vi "VIR.vi"(8 "Stopp":bool, 10 "SLOT":i32=100 min=0 max=999 step=100, 11 "USB":i32) -> ()   [LabVIEW 2020]
doc: "This VI provides a GUI for SLM modules. It implements an abstract module interface, where callers provide the only necessary and sufficient information for callee modules via the datafields USB, SLOT and Stopp. All module intern information are handled hidden by the module. Thereby, a caller must not \"know\" about such internals."
panel:
  in  "Trigger Level":dbl caption="Trigger Level [V]"
  in  "Trigger Source":u16(ring) items=["80 MHz (int.)", "40 MHz (int.)", "20 MHz (int.)", "10 MHz (int.)", " 5 MHz (int.)", " 2.5 MHz (int.)", "rising  edge (ext.)", "falling edge (ext.)"]
  in  "Fan Running":bool
  in  "ZeroBtn":bool caption="Boolean"
  in  "Pulsed Mode":bool
  in  "Intensity":sgl min=0 max=100 step=1 format="%.1f"
  out "Device Type":string
  in  "Frequency":u16(ring) items=["80 MHz (int.)", "40 MHz (int.)", "20 MHz (int.)", "10 MHz (int.)", " 5 MHz (int.)", " 2.5 MHz (int.)", "rising  edge (ext.)", "falling edge (ext.)"]
  # "%"
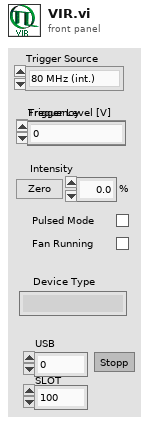
[diagram p1: front panel]
types:
  T1 = enum8{"Enabled", "Disabled", "Disabled and Grayed Out"}
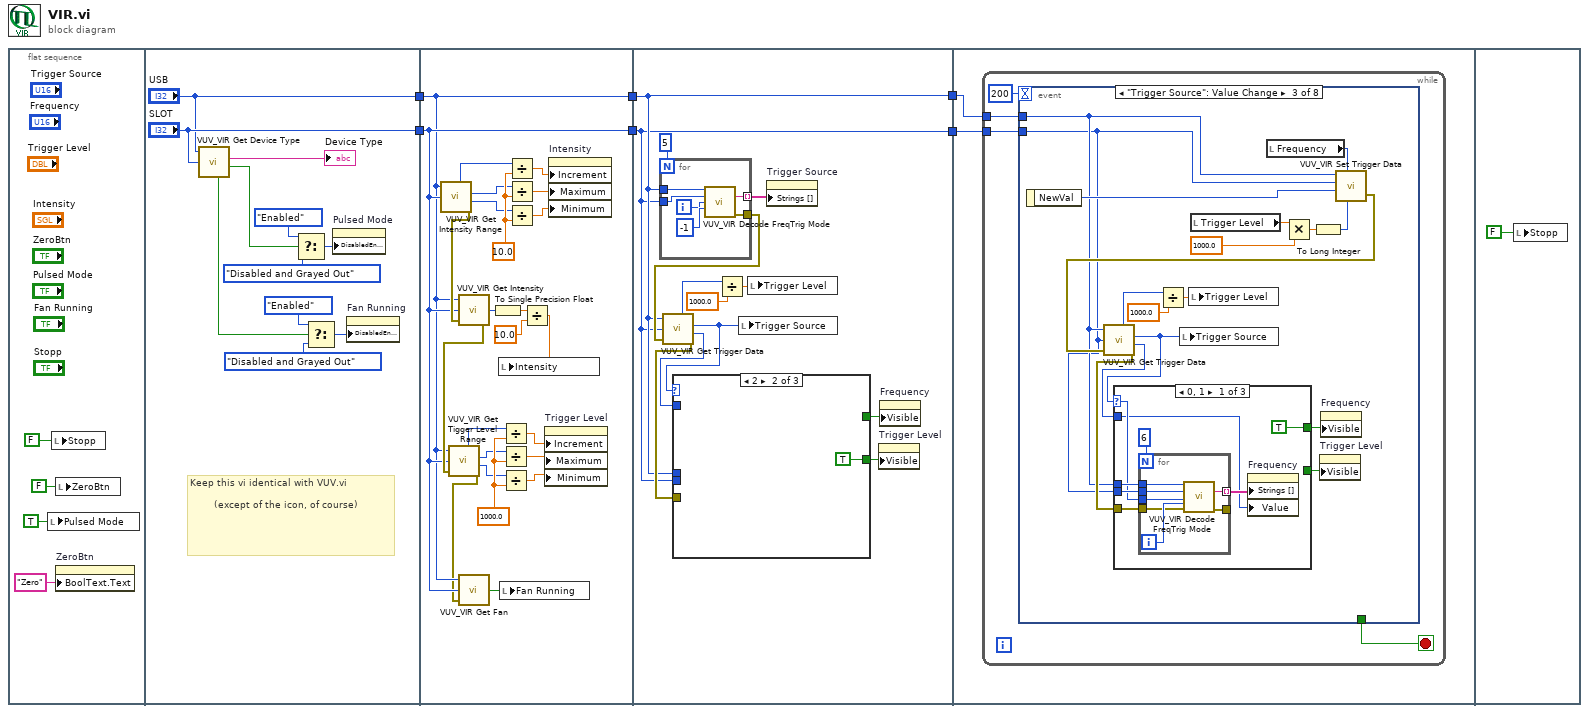
[diagram p0: block diagram]
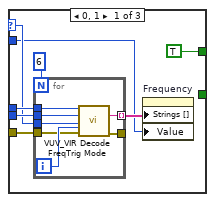
[diagram p2: hidden frame]
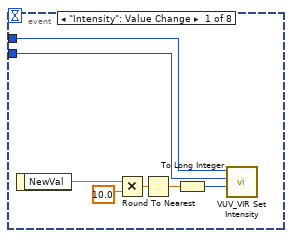
[diagram p4: hidden frame]
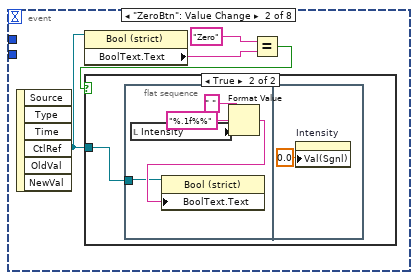
[diagram p5: hidden frame]
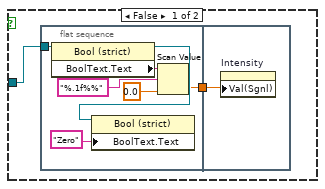
[diagram p6: hidden frame]
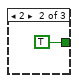
[diagram p7: hidden frame]
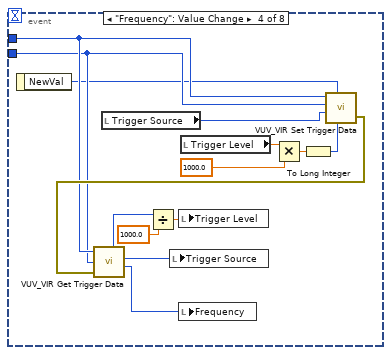
[diagram p9: hidden frame]
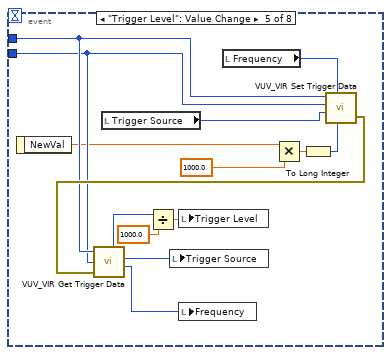
[diagram p10: hidden frame]
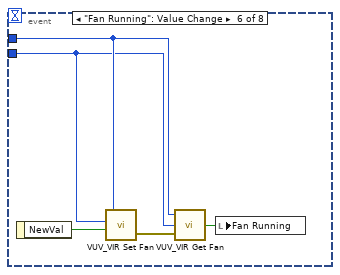
[diagram p11: hidden frame]
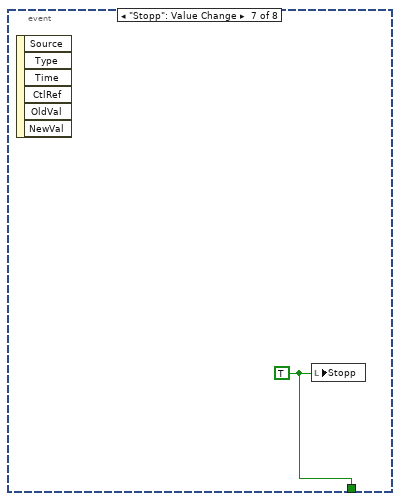
[diagram p12: hidden frame]
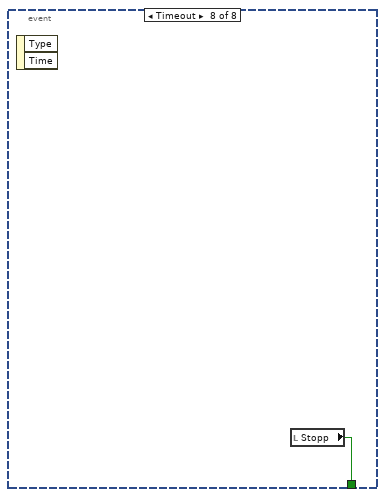
[diagram p13: hidden frame]
diagram:
  n1 = flat-sequence {
    tunnel: ["USB"] -> w6
    tunnel: ["SLOT"] -> w5
    tunnel: w6 -> [w24]
    tunnel: [w24] -> w4
    tunnel: w5 -> [w25]
    tunnel: [w25] -> w3
    tunnel: w4 -> [w47]
    tunnel: w3 -> [w46]
    tunnel: [w47] -> w2
    tunnel: [w46] -> w1
    tunnel: w2 -> [w81]
    tunnel: w1 -> [w82]
    frame #0 {
      n2 = local write "Pulsed Mode"(TRUE ("Pulsed Mode")) -> ()
      n3 = local write "Stopp"(FALSE ("Stopp")) -> ()
      n4 = local write "ZeroBtn"(FALSE ("ZeroBtn")) -> ()
      n5 = property on="ZeroBtn" class="Bool (strict)"("BoolText.Text"="Zero" ("Boolean Text.Text")) -> ()  [unwired: 2 in, 2 out]
    }
    frame #1 {
      # "Keep this vi identical with VUV.vi\n\n        (except of the icon, of course)"
      n6 = call "VUV_VIR Get Device Type.vi"("DevIdx"="USB", "SlotId"="SLOT") -> ("DeviceType"=→"Device Type":string, "OptCW"=w21:bool, "OptFanSwitch"=w14:bool)  [unwired: 1 in, 2 out]
      n7 = Select(t=T1."Enabled" ("Disabled"), s=w21, f=T1."Disabled and Grayed Out" ("Disabled")) -> (s? t:f=w18:T1)
      n8 = Select(t=T1."Enabled" ("Disabled"), s=w14, f=T1."Disabled and Grayed Out" ("Disabled")) -> (s? t:f=w15:T1)
      n9 = property on="Pulsed Mode" class="Bool (strict)"("DisabledEnum"=w18) -> ()  [unwired: 2 in, 2 out]
      n10 = property on="Fan Running" class="Bool (strict)"("DisabledEnum"=w15) -> ()  [unwired: 2 in, 2 out]
    }
    frame #2 {
      w30 = 1000.0
      w45 = 10.0
      n11 = call "VUV_VIR Get Intensity Range.vi"("DevIdx"=w24, "SlotId"=w25) -> ("UpperIntens"=w44:i32, "LowerIntens"=w42:i32, "error out"=w34:errorcluster, "ResolIntens"=w40:i32)  [unwired: 1 in, 1 out]
      n12 = call "VUV_VIR Get Intensity.vi"("error in (no error)"=w34, "SlotId"=w25, "DevIdx"=w24) -> ("error out"=w33:errorcluster, "Intensity"=w38:i32)  [unwired: 1 out]
      n13 = call "VUV_VIR Get Tigger Level Range.vi"("DevIdx"=w24, "SlotId"=w25, "error in (no error)"=w33) -> ("UpperTL"=w28:i32, "LowerTL"=w27:i32, "error out"=w23:errorcluster, "ResolTL"=w29:i32)  [unwired: 1 out]
      n14 = call "VUV_VIR Get Fan.vi"("error in (no error)"=w23, "SlotId"=w25, "DevIdx"=w24) -> ("FanRunning"=w26:bool)  [unwired: 2 out]
      n15 = To Single Precision Float(number=w38) -> (single precision float=w36:sgl)
      n16 = local write "Fan Running"(w26) -> ()
      n17 = Divide(x=w29, y=w30) -> (x/y=w32:dbl)
      n18 = Divide(x=w28, y=w30) -> (x/y=w31:dbl)
      n19 = Divide(x=w27, y=w30) -> (x/y=w22:dbl)
      n20 = Divide(x=w40, y=w45) -> (x/y=w39:dbl)
      n21 = Divide(x=w44, y=w45) -> (x/y=w43:dbl)
      n22 = Divide(x=w42, y=w45) -> (x/y=w41:dbl)
      n23 = Divide(x=w36, y=sgl 10.0) -> (x/y=w37:sgl)
      n24 = local write "Intensity"(w37) -> ()
      n25 = property on="Trigger Level" class="DigNum (strict)"("Increment"=w32, "Maximum"=w31, "Minimum"=w22) -> ()  [unwired: 2 in, 2 out]
      n26 = property on="Intensity" class="DigNum (strict)"("Increment"=w39, "Maximum"=w43, "Minimum"=w41) -> ()  [unwired: 2 in, 2 out]
    }
    frame #3 {
      n27 = for {
        N: 5 ("Numeric") -> [_]
        tunnel: w47 -> [w80]
        tunnel: w46 -> [w79]
        tunnel: [w76] -> w57 mode=indexing
        tunnel: [w75] -> w56
        i -> [w77]
        n28 = call "VUV_VIR Decode FreqTrig Mode.vi"("DevIdx"=w80, "SlotId"=w79, "MainTrigSrcIdx"=w77, "MainFreqDivIdx"=-1) -> ("MainFreqTrig"=w76:string, "error out"=w75:errorcluster)  [unwired: 6 in, 4 out]
      }
      n29 = call "VUV_VIR Get Trigger Data.vi"("DevIdx"=w47, "SlotId"=w46, "error in (no error)"=w56) -> ("MainTrigSrcIdx"=w54:i32, "MainFreqDivIdx"=w52:i32, "error out"=w55:errorcluster, "TrigLevel"=w51:i32)  [unwired: 1 out]
      n30 = case shown="2" w54 {
        selector: w54 -> [w62 _ _]
        tunnel: w47 -> [w65 _ _]
        tunnel: w46 -> [w64 _ _]
        tunnel: w55 -> [w63 _ _]
        tunnel: [TRUE _ _] -> w53
        tunnel: w52 -> [w59 _ _]
        tunnel: [_ TRUE _] -> w48
        frame 0, 1 {
          n31 = for {
            N: 6 ("Numeric") -> [_]
            tunnel: w65 -> [w73]
            tunnel: w64 -> [w72]
            tunnel: [w71] -> w61 mode=indexing
            tunnel: [w70] -> _
            tunnel: w63 -> [w68]
            tunnel: w62 -> [w67]
            i -> [w69]
            n32 = call "VUV_VIR Decode FreqTrig Mode.vi"("DevIdx"=w73, "SlotId"=w72, "MainTrigSrcIdx"=w67, "MainFreqDivIdx"=w69, "error in (no error)"=w68) -> ("MainFreqTrig"=w71:string, "error out"=w70:errorcluster)  [unwired: 5 in, 4 out]
          }
          n33 = property on="Frequency" class="Ring (strict)"("Strings []"=w61, "Value"=w59) -> ()  [unwired: 2 in, 2 out]
        }
        frame 2 {
        }
        frame Default {
        }
      }
      n34 = Divide(x=w51, y=1000.0) -> (x/y=w50:dbl)
      n35 = local write "Trigger Source"(w54) -> ()
      n36 = local write "Trigger Level"(w50) -> ()
      n37 = property on="Trigger Source" class="Ring (strict)"("Strings []"=w57) -> ()  [unwired: 2 in, 2 out]
      n38 = property on="Trigger Level" class="DigNum (strict)"("Visible"=w48) -> ()  [unwired: 2 in, 2 out]
      n39 = property on="Frequency" class="Ring (strict)"("Visible"=w53) -> ()  [unwired: 2 in, 2 out]
    }
    frame #4 {
      n40 = while {
        tunnel: w82 -> [w86]
        tunnel: w81 -> [w85]
        stop <- w83 stop-if-true
        n41 = event shown="[2] \"Trigger Source\": Value Change" {
          selector: _ -> [_ _ _ _ _ _ _ _]
          dyn-events: _ -> [_ _ _ _ _ _ _ _]
          timeout: 200 -> [_ _ _ _ _ _ _ _]
          tunnel: w86 -> [w88 _ w115 w151 w166 w176 _ _]
          tunnel: w85 -> [w87 _ w116 w152 w167 w177 _ _]
          tunnel: [_ _ _ _ _ _ w181 w182] -> w83
          event "Intensity": Value Change {
            n42 = event-data() -> ("NewVal"=w89:sgl)  [unwired: 1 in]
            n43 = Multiply(x=w89, y=sgl 10.0) -> (x*y=w93:sgl)
            n44 = Round To Nearest(number=w93) -> (nearest integer value=w91:sgl)
            n45 = To Long Integer(number=w91) -> (32bit integer=w92:i32)
            n46 = call "VUV_VIR Set Intensity.vi"("Intensity"=w92, "SlotId"=w88, "DevIdx"=w87) -> ()  [unwired: 1 in, 2 out]
          }
          event "ZeroBtn": Value Change {
            n47 = event-data() -> ("CtlRef"=w94:refnum<vi>)  [unwired: 1 in, 5 out]
            n48 = property class="Bool (strict)"(reference=w94) -> ("BoolText.Text"=w96:string)  [unwired: 1 in, 2 out]
            n49 = Equal?(x="Zero" ("Boolean Text.Text"), y=w96) -> (x = y?=w95:bool)
            n50 = case shown="True" w95 {
              tunnel: w94 -> [w99 w108]
              frame False {
                n51 = flat-sequence {
                  tunnel: w99 -> [w106]
                  tunnel: [w101] -> w98
                  tunnel: w98 -> [w107]
                  frame #0 {
                    n52 = property class="Bool (strict)"(reference=w106) -> (reference out=w103:refnum<vi>, "BoolText.Text"=w105:string)  [unwired: 1 in, 1 out]
                    n53 = property class="Bool (strict)"(reference=w103, "BoolText.Text"="Zero" ("Boolean Text.Text")) -> ()  [unwired: 1 in, 2 out]
                    n54 = Scan Value(string=w105, format string="%.1f%%", default (0 dbl)=0.0) -> (value=w101:dbl)  [unwired: 1 out]
                  }
                  frame #1 {
                    n55 = property on="Intensity" class="DigNum (strict)"("Val(Sgnl)"=w107) -> ()  [unwired: 2 in, 2 out]
                  }
                }
              }
              frame True {
                n56 = flat-sequence {
                  tunnel: w108 -> [w109]
                  frame #0 {
                    n57 = local read "Intensity"() -> (w111:sgl)
                    n58 = Format Value(string ("")=" ", format string="%.1f%%", value (0)=w111) -> (output string=w110:string)
                    n59 = property class="Bool (strict)"(reference=w109, "BoolText.Text"=w110) -> ()  [unwired: 1 in, 2 out]
                  }
                  frame #1 {
                    n60 = property on="Intensity" class="DigNum (strict)"("Val(Sgnl)"=sgl 0.0 ("Intensity")) -> ()  [unwired: 2 in, 2 out]
                  }
                }
              }
            }
          }
          event "Trigger Source": Value Change {
            n61 = event-data() -> ("NewVal"=w131:u16)  [unwired: 1 in]
            n62 = local read "Trigger Level"() -> (w129:dbl)
            n63 = local read "Frequency"() -> (w130:u16)
            n64 = Multiply(x=w129, y=1000.0) -> (x*y=w127:dbl)
            n65 = To Long Integer(number=w127) -> (32bit integer=w126:i32)
            n66 = call "VUV_VIR Set Trigger Data.vi"("TrigLevel"=w126, "MainFreqDivIdx"=w130, "MainTrigSrcIdx"=w131, "SlotId"=w115, "DevIdx"=w116) -> ("error out"=w119:errorcluster)  [unwired: 1 in, 1 out]
            n67 = call "VUV_VIR Get Trigger Data.vi"("DevIdx"=w116, "SlotId"=w115, "error in (no error)"=w119) -> ("MainTrigSrcIdx"=w120:i32, "MainFreqDivIdx"=w117:i32, "error out"=w118:errorcluster, "TrigLevel"=w122:i32)  [unwired: 1 out]
            n68 = case shown="0, 1" w120 {
              selector: w120 -> [w135 _ _]
              tunnel: w116 -> [w138 _ _]
              tunnel: w115 -> [w137 _ _]
              tunnel: w118 -> [w136 _ _]
              tunnel: [TRUE _ _] -> w121
              tunnel: w117 -> [w132 _ _]
              tunnel: [_ TRUE _] -> w125
              frame 0, 1 {
                n69 = for {
                  N: 6 ("Numeric") -> [_]
                  tunnel: w138 -> [w146]
                  tunnel: w137 -> [w145]
                  tunnel: [w144] -> w134 mode=indexing
                  tunnel: [w143] -> _
                  tunnel: w136 -> [w141]
                  tunnel: w135 -> [w140]
                  i -> [w142]
                  n70 = call "VUV_VIR Decode FreqTrig Mode.vi"("DevIdx"=w146, "SlotId"=w145, "MainTrigSrcIdx"=w140, "MainFreqDivIdx"=w142, "error in (no error)"=w141) -> ("MainFreqTrig"=w144:string, "error out"=w143:errorcluster)  [unwired: 5 in, 4 out]
                }
                n71 = property on="Frequency" class="Ring (strict)"("Strings []"=w134, "Value"=w132) -> ()  [unwired: 2 in, 2 out]
              }
              frame 2 {
              }
              frame Default {
              }
            }
            n72 = Divide(x=w122, y=1000.0) -> (x/y=w123:dbl)
            n73 = local write "Trigger Source"(w120) -> ()
            n74 = local write "Trigger Level"(w123) -> ()
            n75 = property on="Trigger Level" class="DigNum (strict)"("Visible"=w125) -> ()  [unwired: 2 in, 2 out]
            n76 = property on="Frequency" class="Ring (strict)"("Visible"=w121) -> ()  [unwired: 2 in, 2 out]
          }
          event "Frequency": Value Change {
            n77 = event-data() -> ("NewVal"=w150:u16)  [unwired: 1 in]
            n78 = local read "Trigger Source"() -> (w149:u16)
            n79 = local read "Trigger Level"() -> (w161:dbl)
            n80 = Multiply(x=w161, y=1000.0) -> (x*y=w159:dbl)
            n81 = To Long Integer(number=w159) -> (32bit integer=w158:i32)
            n82 = call "VUV_VIR Set Trigger Data.vi"("TrigLevel"=w158, "MainFreqDivIdx"=w150, "MainTrigSrcIdx"=w149, "SlotId"=w151, "DevIdx"=w152) -> ("error out"=w153:errorcluster)  [unwired: 1 in, 1 out]
            n83 = call "VUV_VIR Get Trigger Data.vi"("DevIdx"=w152, "SlotId"=w151, "error in (no error)"=w153) -> ("MainTrigSrcIdx"=w154:i32, "MainFreqDivIdx"=w148:i32, "TrigLevel"=w155:i32)  [unwired: 2 out]
            n84 = Divide(x=w155, y=1000.0) -> (x/y=w156:dbl)
            n85 = local write "Trigger Source"(w154) -> ()
            n86 = local write "Trigger Level"(w156) -> ()
            n87 = local write "Frequency"(w148) -> ()
          }
          event "Trigger Level": Value Change {
            n88 = event-data() -> ("NewVal"=w163:dbl)  [unwired: 1 in]
            n89 = local read "Trigger Source"() -> (w165:u16)
            n90 = local read "Frequency"() -> (w162:u16)
            n91 = Multiply(x=w163, y=1000.0) -> (x*y=w174:dbl)
            n92 = To Long Integer(number=w174) -> (32bit integer=w173:i32)
            n93 = call "VUV_VIR Set Trigger Data.vi"("TrigLevel"=w173, "MainFreqDivIdx"=w162, "MainTrigSrcIdx"=w165, "SlotId"=w166, "DevIdx"=w167) -> ("error out"=w168:errorcluster)  [unwired: 1 in, 1 out]
            n94 = call "VUV_VIR Get Trigger Data.vi"("DevIdx"=w167, "SlotId"=w166, "error in (no error)"=w168) -> ("MainTrigSrcIdx"=w169:i32, "MainFreqDivIdx"=w164:i32, "TrigLevel"=w170:i32)  [unwired: 2 out]
            n95 = Divide(x=w170, y=1000.0) -> (x/y=w171:dbl)
            n96 = local write "Trigger Source"(w169) -> ()
            n97 = local write "Trigger Level"(w171) -> ()
            n98 = local write "Frequency"(w164) -> ()
          }
          event "Fan Running": Value Change {
            n99 = event-data() -> ("NewVal"=w180:bool)  [unwired: 1 in]
            n100 = call "VUV_VIR Set Fan.vi"("FanRunning"=w180, "SlotId"=w176, "DevIdx"=w177) -> ("error out"=w178:errorcluster)  [unwired: 1 in, 1 out]
            n101 = call "VUV_VIR Get Fan.vi"("error in (no error)"=w178, "SlotId"=w176, "DevIdx"=w177) -> ("FanRunning"=w179:bool)  [unwired: 2 out]
            n102 = local write "Fan Running"(w179) -> ()
          }
          event "Stopp": Value Change {
            w181 = TRUE ("Value (Signaling)")
            n103 = event-data() -> ()  [unwired: 1 in, 6 out]
            n104 = local write "Stopp"(w181) -> ()
          }
          event Timeout {
            n105 = event-data() -> ()  [unwired: 1 in, 2 out]
            n106 = local read "Stopp"() -> (w182:bool)
          }
        }
      }
    }
    frame #5 {
      n107 = local write "Stopp"(FALSE ("Stopp")) -> ()
    }
  }
